vi "VNA_Easy_Initialize.vi"(8 "error in (no error)":errorcluster, 10 "Power (dbm)":dbl=-10.0, 11 "VISA Refnum in":refnum<visa-resource-name>) -> (0 "error out":errorcluster, 3 "VISA Refnum out":refnum<visa-resource-name>)   [LabVIEW 2020]
uses:
  <instrlib>/Agilent 87XX Series/Agilent 87XX Series.lvlib
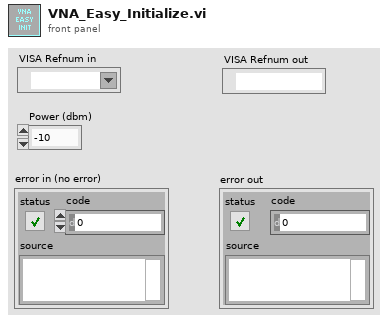
[diagram p1: front panel]
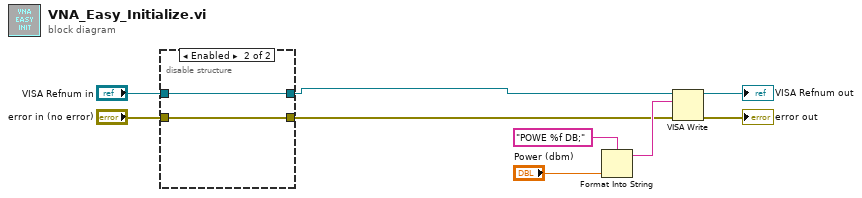
[diagram p0: block diagram]
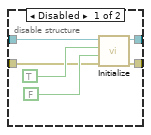
[diagram p2: hidden frame]
diagram:
  n1 = disable-structure shown="Enabled" {
    disable-tunnel: [w13 w17] -> w2
    disable-tunnel: [w12 w16] -> w1
    disable-tunnel: "VISA Refnum in" -> [w11 w17]
    disable-tunnel: "error in (no error)" -> [w10 w16]
    frame Disabled {
      n2 = call <instrlib>:"Initialize.vi"("error in (no error)"=w10, "reset"=FALSE, "ID query"=TRUE, "VISA resource name"=w11) -> ("error out"=w12:errorcluster, "VISA resource name out"=w13:refnum<visa-resource-name>)  [unwired: 6 in]
    }
    frame Enabled {
    }
  }
  n3 = Format Into String(format string="POWE %f DB;", "Power (dbm)") -> (resulting string=w5:string)  [unwired: 2 in, 1 out]
  n4 = VISA Write(VISA resource name=w2, write buffer=w5, error in (no error)=w1) -> (VISA resource name out=→"VISA Refnum out":refnum<visa-resource-name>, error out=→"error out":errorcluster)  [unwired: 1 out]
